vi "createParagraph.vi"(8 "error in (no error)":errorcluster, 9 "Style":refnum<class "Style.lvclass">, 10 "Text":string, 11 "MS-Word in":refnum<class "MS-Word.lvclass">) -> (0 "error out":errorcluster, 3 "MS-Word out":refnum<class "MS-Word.lvclass">)   [LabVIEW 2017, in "LabVIEW NPOI.lvlib" / "MS-Word.lvclass"]
uses:
  MS-Word.lvclass
  Styles/Style/Style.lvclass
  MS-Word.lvclass/MS-Word.ctl
  C:/Users/Neo/Desktop/Dev_Tools_BR/LabVIEW_NPOI/lib/NPOI 2.1.1/NPOI.OOXML.dll
  lib/NPOI 2.1.1/NPOI.OOXML.dll
panel:
  out "Text 2":string
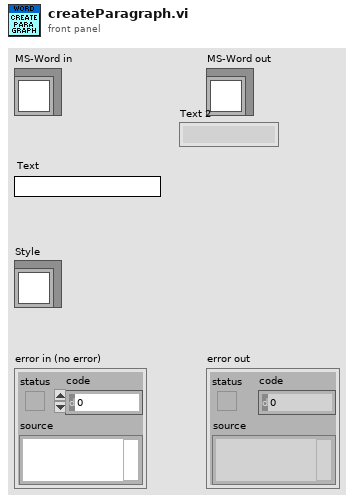
[diagram p1: front panel]
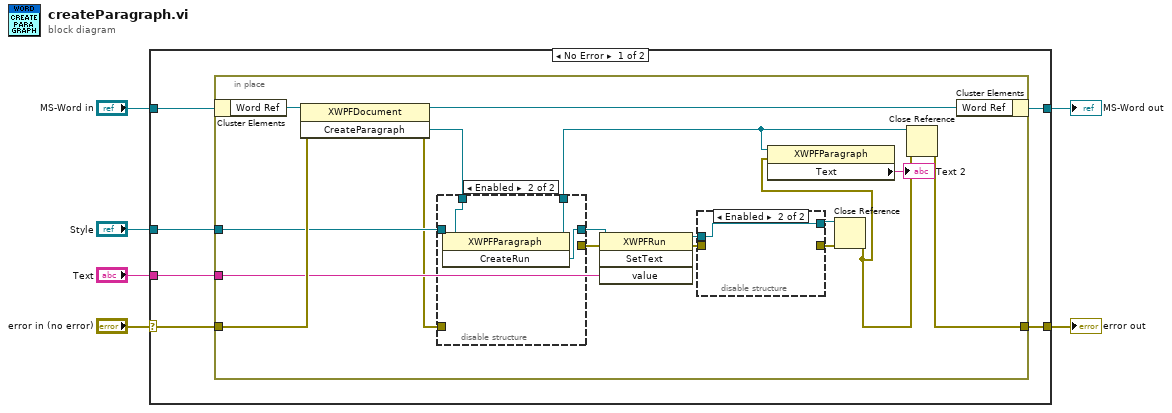
[diagram p0: block diagram]
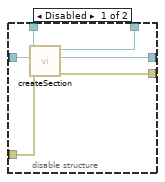
[diagram p2: hidden frame]
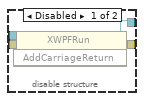
[diagram p3: hidden frame]
diagram:
  n1 = case shown="No Error" "error in (no error)" {
    selector: "error in (no error)" -> [w10 w45]
    tunnel: [w9 w45] -> w5
    tunnel: [w12 w44] -> w3
    tunnel: "MS-Word in" -> [w11 w44]
    tunnel: "Style" -> [w8 _]
    tunnel: "Text" -> [w7 _]
    frame No Error {
      n2 = in-place {
        in-place-border: w10 -> [w28]
        in-place-border: [w17] -> w9
        in-place-border: w8 -> [w26]
        in-place-border: w7 -> [w23]
        n3 = in-place-cluster #1(w11) -> ("Word Ref"=w29:refnum<k24>)
        n4 = invoke class="XWPFDocument" method="CreateParagraph"(reference=w29, error in=w28) -> (reference out=w27:refnum<k24>, error out=w16:errorcluster, "CreateParagraph"=w18:refnum<k24>)  [unwired: 1 in]
        n5 = disable-structure shown="Enabled" {
          disable-tunnel: w26 -> [w35 _]
          disable-tunnel: [w34 w36] -> w25
          disable-tunnel: [w33 _] -> w24
          disable-tunnel: w18 -> [w32 w38]
          disable-tunnel: w16 -> [w31 _]
          disable-tunnel: [w30 w37] -> w15
          frame Disabled {
            n6 = call "createSection.vi"("error in (no error)"=w31, "Style"=w35, "Paragraph in"=w32) -> ("error out"=w33:errorcluster, "Section out"=w34:refnum<k24>, "Paragraph out"=w30:refnum<k24>)  [unwired: 6 in]
          }
          frame Enabled {
            n7 = invoke class="XWPFParagraph" method="CreateRun"(reference=w38) -> (reference out=w37:refnum<k24>, "CreateRun"=w36:refnum<k24>)  [unwired: 2 in, 1 out]
          }
        }
        n8 = invoke class="XWPFRun" method="SetText"(reference=w25, error in=w24, "value"=w23) -> (reference out=w22:refnum<k24>, error out=w21:errorcluster)  [unwired: 1 in, 2 out]
        n9 = disable-structure shown="Enabled" {
          disable-tunnel: w22 -> [w42 w43]
          disable-tunnel: w21 -> [w41 _]
          disable-tunnel: [w40 w43] -> w20
          disable-tunnel: [w39 _] -> w19
          frame Disabled {
            n10 = invoke class="XWPFRun" method="AddCarriageReturn"(reference=w42, error in=w41) -> (reference out=w40:refnum<k24>, error out=w39:errorcluster)  [unwired: 1 in, 1 out]
          }
          frame Enabled {
          }
        }
        n11 = Close Reference(reference=w20, error in (no error)=w19) -> (error out=w13:errorcluster)
        n12 = property class="XWPFParagraph"(reference=w15, error in=w13) -> ("Text"=→"Text 2":string)  [unwired: 2 out]
        n13 = Close Reference(reference=w15, error in (no error)=w13) -> (error out=w17:errorcluster)
        n14 = in-place-cluster #1("Word Ref"=w27) -> (w12:refnum<class "MS-Word.lvclass">)
      }
    }
    frame Error {
    }
  }
  "error out" <- w5
  "MS-Word out" <- w3
